vi "service_error_parse.vi"(3 "error in (no error)":errorcluster, 5 "Reply":string="\u0000\u0000\u0000\u0000\u0000") -> (0 "error out":errorcluster, 1 "OK?":bool, 2 "Log string":string)   [LabVIEW 2016]
doc: "Parses a message into a service error"
uses:
  std_msgs/subs/parse_u8_scalar.vi
panel:
  out "Error Code":i32
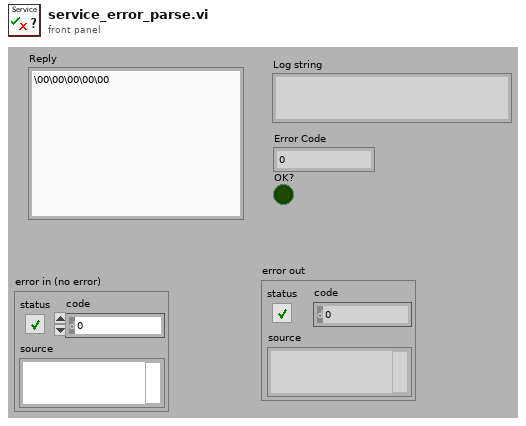
[diagram p1: front panel]
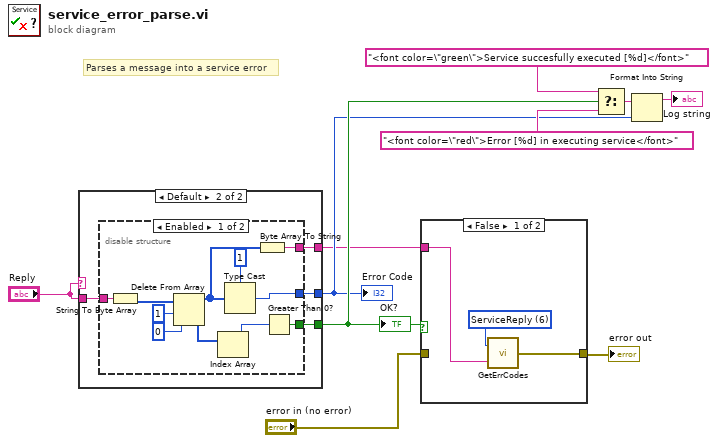
[diagram p0: block diagram]
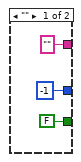
[diagram p3: hidden frame]
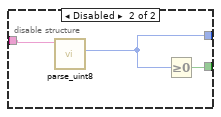
[diagram p4: hidden frame]
diagram:
  # "Parses a message into a service error"
  n1 = case shown="Default" "Reply" {
    tunnel: "Reply" -> [_ w17]
    tunnel: [-1 ("length") w16] -> w4
    tunnel: [FALSE w15] -> w7
    tunnel: ["" ("string") w14] -> w1
    frame "" {
    }
    frame Default {
      n2 = disable-structure shown="Enabled" {
        disable-tunnel: w17 -> [w28 w31]
        disable-tunnel: [w23 w29] -> w16
        disable-tunnel: [w22 w30] -> w15
        disable-tunnel: [w18 _] -> w14
        frame Enabled {
          n3 = String To Byte Array(string=w28) -> (unsigned byte array=w27:u8[])
          n4 = Delete From Array(array=w27, length=1, index=0) -> (deleted portion=w21:u8[], array with subset deleted=w19:u8[])
          n5 = Index Array(array=w21) -> (element=w20:u8)  [unwired: 1 in]
          n6 = Type Cast(type=1 ("length"), x=w19) -> (*(type *) &x=w23:i32)
          n7 = Byte Array To String(unsigned byte array=w19) -> (string=w18:string)
          n8 = Greater Than 0?(x=w20) -> (x > 0?=w22:bool)
        }
        frame Disabled {
          n9 = call-poly "parse_uint8.vi"("msg in"=w31) -> ("number"=w29:u8)  [unwired: 4 in, 2 out]
          n10 = Greater Or Equal To 0?(x=w29) -> (x >= 0?=w30:bool)
        }
      }
    }
  }
  "Error Code" <- w4
  "OK?" <- w7
  n11 = case shown="False" w7 {
    tunnel: [w32 w35] -> w8
    tunnel: "error in (no error)" -> [_ w35]
    tunnel: w1 -> [w33 _]
    frame False {
      w34 = u16 6 items=["TopicReadTimeout", "Read=SS", "GetQueueErr", "NoMaster", "Write=PS", "Unparse", "ServiceReply"] ("Error")
      n12 = call "GetErrCodes.vi"("Added Text"=w33, "Error"=w34) -> ("Error"=w32:errorcluster)
    }
    frame True {
    }
  }
  "error out" <- w8
  n13 = Select(t="<font color=\"green\">Service succesfully executed [%d]</font>" ("Text to add"), s=w7, f="<font color=\"red\">Error [%d] in executing service</font>" ("Text to add")) -> (s? t:f=w3:string)
  n14 = Format Into String(format string=w3, w4) -> (resulting string=→"Log string":string)  [unwired: 2 in, 1 out]
